vi "test Verify AND Combos.vi"(8 "error in":errorcluster, 11 "Testing Approval Tests in":refnum<class "VITester Extension Tests.lvclass">) -> (0 "error out":errorcluster, 3 "Testing Approval Tests out":refnum<class "VITester Extension Tests.lvclass">)   [LabVIEW 2026, in "VITester Extension Tests.lvclass"]
uses:
  VITester Extension Tests.lvclass
  C:/Program Files/National Instruments/LabVIEW 2026/vi.lib/Addons/_JKI Toolkits/VI Tester/TestCase.llb/TestCase.lvclass
  c9a13bd5-c875-47b0-8404-7b4d8af749e1.vi
  Source/Extensions/VITester.Extension/VITester.Extension.lvlib
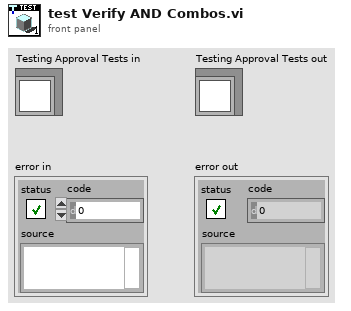
[diagram p1: front panel]
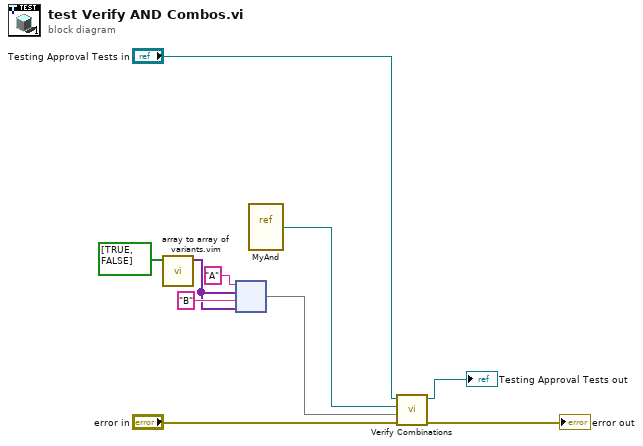
[diagram p0: block diagram]
diagram:
  n1 = call "array to array of variants.vim"("Array in"=bool[] [TRUE, FALSE]) -> ("Array out"=w3:variant[])  [unwired: 10 in]
  n2 = node ("Build Map")("A" ("key"), w3, "B" ("key"), w3) -> (w2:map{string, variant[]})
  n3 = vi-ref "MyAnd.vi"() -> (w1:refnum<vi>)
  n4 = call "Verify Combinations.vi"("error in"="error in", "ctl label -> value var[]"=w2, "VI Refnum"=w1, "TestCase in"="Testing Approval Tests in") -> ("error out"=→"error out":errorcluster, "TestCase out"=→"Testing Approval Tests out":refnum<class "VITester Extension Tests.lvclass">)  [unwired: 6 in]
